vi "Configure Autozero.vi"(8 "error in (no error)":errorcluster, 10 "Autozero  (0: On)":u16(ring) items=["On", "Off", "Once"], 11 "VISA resource name":refnum<visa-resource-name>) -> (0 "error out":errorcluster, 3 "VISA resource name out":refnum<visa-resource-name>)   [LabVIEW 2012, in "Agilent 34401.lvlib"]
doc: "Configures the autozero setting on the instrument. Enabling autozero optimizes the instrument for accuracy, while disabling optimizes for speed."
uses:
  Agilent 34401.lvlib
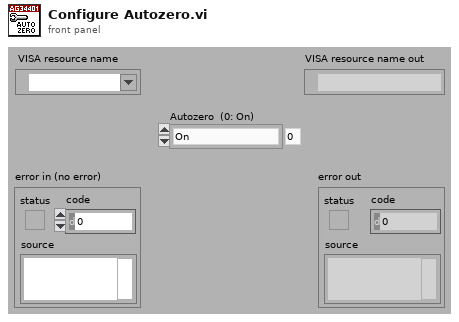
[diagram p1: front panel]
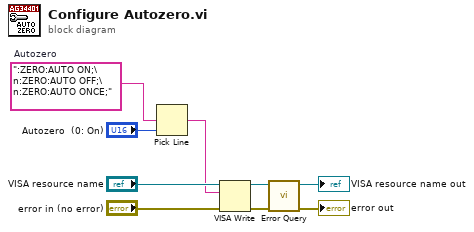
[diagram p0: block diagram]
diagram:
  w1 = ":ZERO:AUTO ON;\n:ZERO:AUTO OFF;\n:ZERO:AUTO ONCE;"  # Autozero
  n1 = Pick Line(multi-line string=w1, line index="Autozero  (0: On)") -> (output string=w3:string)  [unwired: 1 in]
  n2 = VISA Write(VISA resource name="VISA resource name", write buffer=w3, error in (no error)="error in (no error)") -> (VISA resource name out=w5:refnum<visa-resource-name>, error out=w4:errorcluster)  [unwired: 1 out]
  n3 = call "Error Query.vi"("error in (no error)"=w4, "VISA resource name"=w5) -> ("error out"=→"error out":errorcluster, "VISA resource name out"=→"VISA resource name out":refnum<visa-resource-name>)  [unwired: 6 in, 2 out]
